vi "Example of fpPrintScreen.vi"() -> ()   [LabVIEW 2016]
uses:
  <vilib>/Platform/browser.llb/Open URL in Default Browser (path).vi
panel:
  out "Image saved path":path
  in  "Open":bool caption="Open and view saved image"
  in  "PRTSC":bool caption="Press PRTSC or use keyboard shortcut F1 to print screen"
  in  "stop":bool
  # "Hint: use Key Navigation to assign a shortcut to some button"
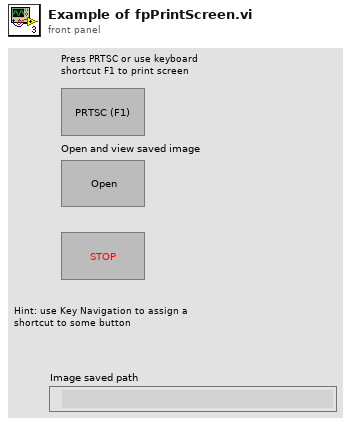
[diagram p1: front panel]
types:
  T1 = enum8{"Enabled", "Disabled", "Disabled and Grayed Out"}
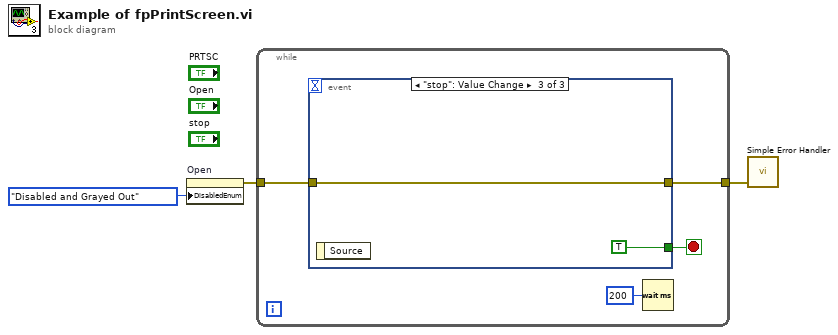
[diagram p0: block diagram]
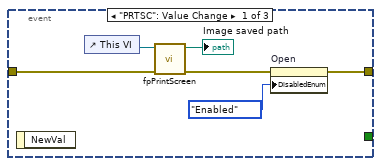
[diagram p2: hidden frame]
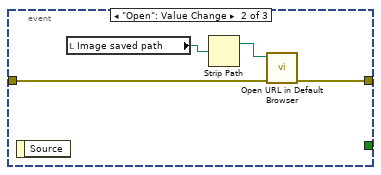
[diagram p3: hidden frame]
diagram:
  n1 = property on="Open" class="Bool"("DisabledEnum"=T1."Disabled and Grayed Out" ("Disabled")) -> (error out=w3:errorcluster)  [unwired: 2 in, 1 out]
  n2 = while {
    tunnel: w3 -> [w5]
    tunnel: [w4] -> w1
    stop <- w6 stop-if-true
    n3 = event shown="[2] \"stop\": Value Change" {
      selector: _ -> [_ _ _]
      dyn-events: _ -> [_ _ _]
      timeout: _ -> [_ _ _]
      tunnel: [_ _ TRUE] -> w6
      tunnel: w5 -> [w9 w15 w18]
      tunnel: [w8 w14 w18] -> w4
      event "PRTSC": Value Change {
        n4 = event-data() -> ()  [unwired: 1 in, 1 out]
        n5 = control-ref of="This VI"() -> (w13:refnum<vi>)
        n6 = call "fpPrintScreen.vi"("error in (no error)"=w9, "VI ref"=w13) -> ("error out"=w10:errorcluster, "image saved path"=→"Image saved path":path)  [unwired: 8 in]
        n7 = property on="Open" class="Bool"(error in=w10, "DisabledEnum"=T1."Enabled" ("Disabled")) -> (error out=w8:errorcluster)  [unwired: 1 in, 1 out]
      }
      event "Open": Value Change {
        n8 = event-data() -> ()  [unwired: 1 in, 1 out]
        n9 = local read "Image saved path"() -> (w17:path)
        n10 = Strip Path(path=w17) -> (stripped path=w16:path)  [unwired: 1 out]
        n11 = call-poly <vilib>:"Open URL in Default Browser.vi"("error in (no error)"=w15, "path"=w16) -> ("error out"=w14:errorcluster)  [unwired: 4 in, 1 out]
      }
      event "stop": Value Change {
        n12 = event-data() -> ()  [unwired: 1 in, 1 out]
      }
    }
    n13 = Wait (ms)(milliseconds to wait=u32 200) -> ()  [unwired: 1 out]
  }
  n14 = call <vilib>:"Simple Error Handler.vi"("error in (no error)"=w1) -> ()  [unwired: 4 in, 5 out]
